vi "Communication Global variables.vi"() -> ()   [LabVIEW 2016]
panel:
  in  "REST Timeout":i32=500
  in  "REST URL":string="http://localhost:5800"
  in  "UDP connection ID":refnum<k16>
  in  "IP address":u32=169558786
  in  "NetworkP_RobotAddress":string="10.27.67.2"
  in  "UDP port":u16=5555
  # "not currently used:"
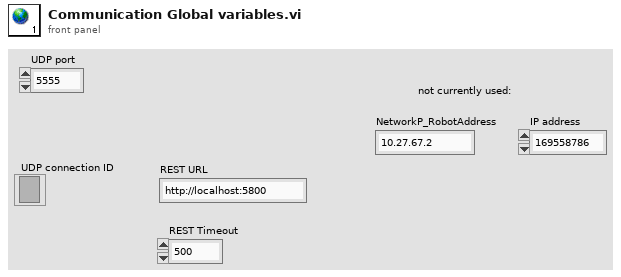
[diagram p1: front panel]
diagram:
